vi "RSNRPZ Set Duty Cycle.vi"(8 "error in (no error)":errorcluster, 9 "Duty Cycle (1.0 %)":dbl=1.0 format="%.2p", 10 "Channel (1)":i32=1, 11 "VISA session":refnum<visa-resource-name> caption="VISA resource name") -> (0 "error out":errorcluster, 3 "dup VISA session":refnum<visa-resource-name> caption="VISA resource name")   [LabVIEW 2010]
doc: "This VI informs the R&S NRP about the duty cycle of the power to be measured. Specifying a duty cycle only makes sense in the ContAv mode where measurements are performed continuously without taking the timing of the signal into account. For this reason, this setting can only be chosen in the local mode when the sensor performs measurements in the ContAv mode.\n\nRemote-control command(s):\nSENS:CORR:DCYC"
uses:
  rsnrpz_32.dll
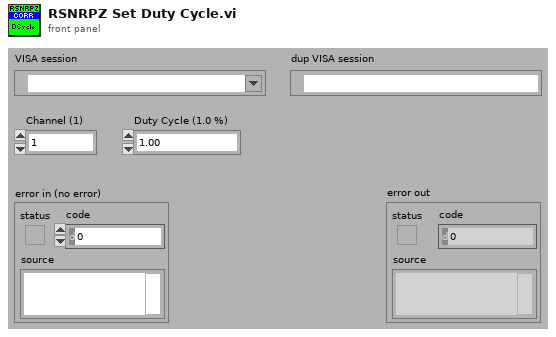
[diagram p1: front panel]
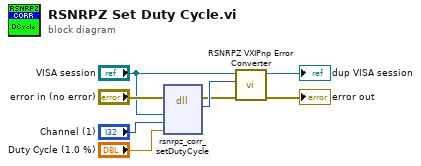
[diagram p0: block diagram]
diagram:
  n1 = dll-call lib="rsnrpz_32.dll" fn="rsnrpz_corr_setDutyCycle"(error in="error in (no error)", "VISA Session"="VISA session", "Channel"="Channel (1)", "Duty Cycle"="Duty Cycle (1.0 %)") -> (error out=w5:errorcluster, "Status"=w8:i32)  [unwired: 5 in, 1 out]
  n2 = call <instrlib>:"RSNRPZ VXIPnp Error Converter.vi"("error in"=w5, "VXIPnp error code"=w8, "VISA session"="VISA session") -> ("error out"=→"error out":errorcluster, "dup VISA session"=→"dup VISA session":refnum<visa-resource-name>)  [unwired: 7 in]
